vi "ROI entry-bundle parameter values.vi"(7 "XYZ_Coordinates":T1[](array[typedef]) {"ROI group ID" format="%#_6f"; "Laser Power (%)" format="%#_6f"; "Zoom" format="%#_6f"; "Frame Size" format="%#_6f"; "Number of lines" format="%#_6f"; "Composite ID" format="%#_6f"; "Angle (deg)" format="%#_6f"; "ROI Time (ns)" format="%#_6f"; "ROI ID" format="%#_6f"; "Pixels in ROI" format="%#_6f"; "ROI index" format="%#_6f"; "Z stop" format="%#_6f"; "Y stop" format="%#_6f"; "X stop" format="%#_6f"; "Z start" format="%#_6f"; "X start" format="%#_6f"; "Y start" format="%#_6f"}, 8 "error in (no error)":errorcluster, 9 "Button Label.Text":string) -> (0 "error out":errorcluster, 3 "AOL_Globals out":T2={"Imaging Protocol"=enum."AOL Z-Stack", "Number of POI"=0, "Number of Miniscans"=0, "Number of Trials"=0, "Number of Cycles "=0, "# Averaged Frames"=0, "Laser power (%)"=0, "Pockels (V)"=0.0, "Acquisition Length (sec)"=0.0, "Fill time (us)"=0.0, "POI Dwell time (us)"=0.0, "Miniscan Dwell time per pixel (us)"=0.0, "PMT 1"=0.0, "PMT 2"=0.0, "Back Apperture (mA)"=0.0, "Frame Size"=0, "Center Frequency"=0.0, "Field of View (norm)"=0.0, "DwellTime (us)"=0.0, "Wavelength (nm)"=0.0, "Zoom"=0.0, "AOL Z"=0.0, "AOL Mode"=enum."Raster", "GridXY"=0.0, "GridZ"=0.0, "TriggerPeriod (sec)"=0.0, "Number of Pixels in Miniscan"=0, "Experiment folder path"=path "", "X centre"=0.0, "Y centre"=0.0, "Angle (degrees)"=0.0, "Plane Mode"=0, "Threshold"=[], "Regenerate Chirps"=FALSE, "Rectangle ROI length (pixels)"=0, "Rectangle ROI height (pixels)"=0, "AOD fill"=4900, "StartupDelay"=0, "Samples Wait after Trigger"=5080, "Slip Cycle"=600000, "Add Cycle"=TRUE, "Functional Mode"=enum."Point", "Z Start"=0.0, "Z Stop"=0.0, "# Planes"=0} {"Plane Mode" items=["XY Plane", "XZ Plane", "YZ Plane", "arbitraryplane"]; "Frame Size" items=["100X100"=100, "128X128"=128, "200X200"=200, "256X256"=256, "512X512"=512, "1024x1024"=1024, "2048x2048"=2048]; "Back Apperture (mA)" format="%#.6g"; "Pockels (V)" format="%#.6g"; "PMT 2" format="%#.6g"; "PMT 1" format="%#.6g"; "Angle (degrees)" format="%#.6g"; "POI Dwell time (us)" format="%#.6g"})   [LabVIEW 2017]
uses:
  Typedefs/Controls/AOL_Globals.ctl
  Typedefs/Imaging Protocols enum.ctl
  Typedefs/Frame Size.ctl
  Typedefs/AOL modes.ctl
  Typedefs/Plane Mode.ctl
  Typedefs/Functional Mode.ctl
  Visualisation/Functional Imaging Viewer/Typedefs/ROI parameters data type.ctl
  <userlib>/_MGI/Application Control/MGI Change Detector/MGI Change Detector (T).vi
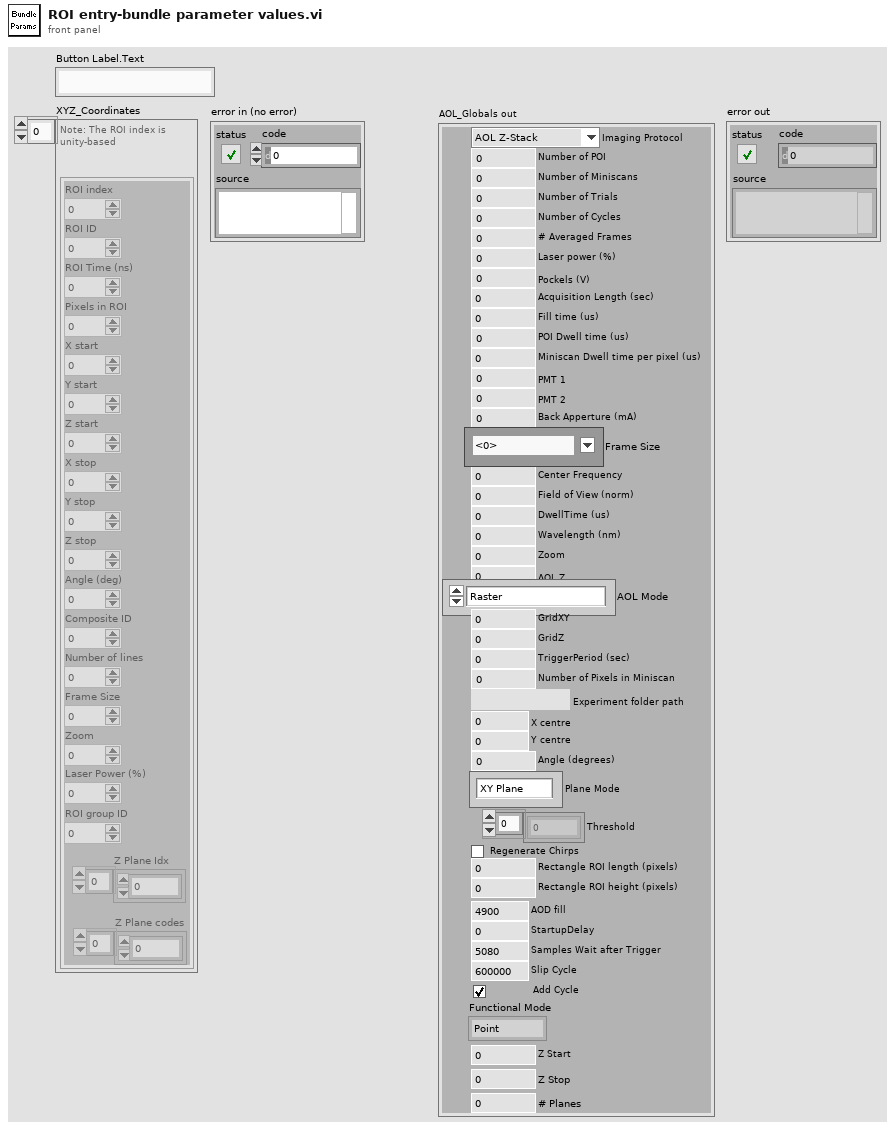
[diagram p1: front panel]
types:
  T1 = typedef "ROI parameters data type.ctl" = cluster{"ROI index":dbl, "ROI ID":dbl, "ROI Time (ns)":dbl, "Pixels in ROI":dbl, "X start":dbl, "Y start":dbl, "Z start":dbl, "X stop":dbl, "Y stop":dbl, "Z stop":dbl, "Angle (deg)":dbl, "Composite ID":dbl, "Number of lines":dbl, "Frame Size":dbl, "Zoom":dbl, "Laser Power (%)":dbl, "ROI group ID":dbl, "Z Plane Idx":i32[], "Z Plane codes":i32[]}
  T2 = typedef "AOL_Globals.ctl" = cluster{"Imaging Protocol":T3, "Number of POI":u16, "Number of Miniscans":u16, "Number of Trials":u16, "Number of Cycles ":u64, "# Averaged Frames":u16, "Laser power (%)":u8, "Pockels (V)":dbl, "Acquisition Length (sec)":dbl, "Fill time (us)":dbl, "POI Dwell time (us)":dbl, "Miniscan Dwell time per pixel (us)":dbl, "PMT 1":dbl, "PMT 2":dbl, "Back Apperture (mA)":dbl, "Frame Size":T4, "Center Frequency":dbl, "Field of View (norm)":dbl, "DwellTime (us)":dbl, "Wavelength (nm)":dbl, "Zoom":dbl, "AOL Z":dbl, "AOL Mode":T5, "GridXY":dbl, "GridZ":dbl, "TriggerPeriod (sec)":dbl, "Number of Pixels in Miniscan":u16, "Experiment folder path":path, "X centre":dbl, "Y centre":dbl, "Angle (degrees)":dbl, "Plane Mode":T6, "Threshold":u16[], "Regenerate Chirps":bool, "Rectangle ROI length (pixels)":u16, "Rectangle ROI height (pixels)":u16, "AOD fill":u16, "StartupDelay":i32, "Samples Wait after Trigger":u16, "Slip Cycle":u32, "Add Cycle":bool, "Functional Mode":T7, "Z Start":dbl, "Z Stop":dbl, "# Planes":i32}
  T3 = typedef "Imaging Protocols enum.ctl" = enum16{"AOL Z-Stack", "Motor Z Stack", "Functional Acquisition", "Single Plane Acquisition", "Volume Acquisition", "Live Imaging", "Live Plane Imaging", "Live Volume Imaging"}
  T4 = typedef "Frame Size.ctl" = u16
  T5 = typedef "AOL modes.ctl" = enum16{"Raster", "Structural", "Pointing", "Mini Scan", "Alignment"}
  T6 = typedef "Plane Mode.ctl" = u16
  T7 = typedef "Functional Mode.ctl" = enum16{"Point", "Line", "Patch", "Plane", "Volume"}
  T8 = typedef "ROI ID Enum.ctl" = enum16{"Point", "MiniScan", "Comp. MiniScan", "Rectangle", "Comp. volume", "Arb. plane point", "None"}
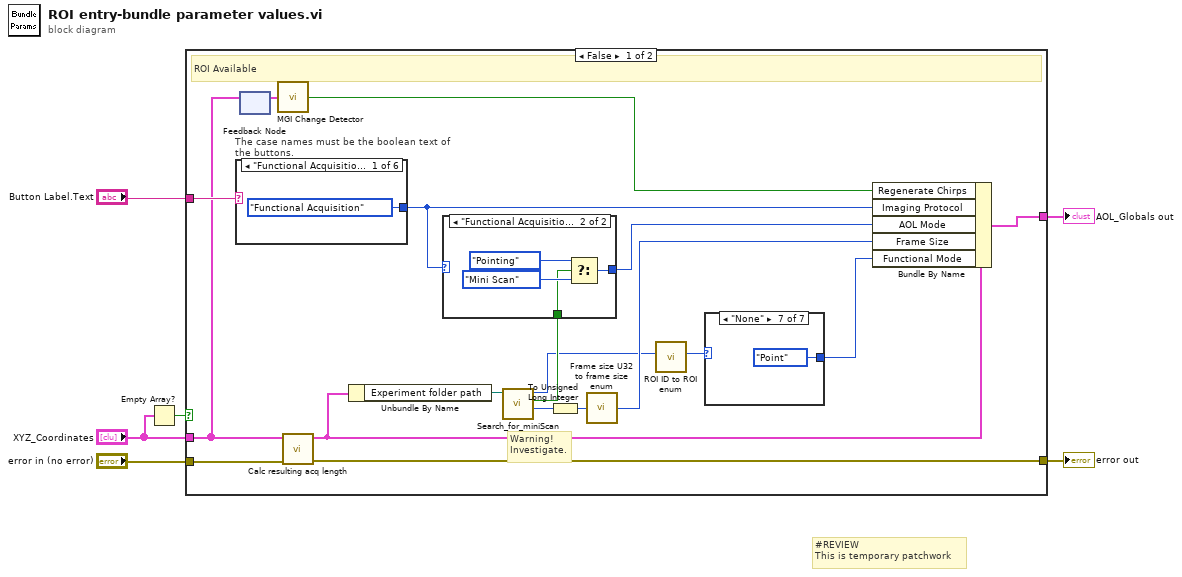
[diagram p0: block diagram]
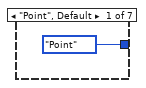
[diagram p2: hidden frame]
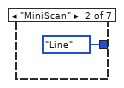
[diagram p3: hidden frame]
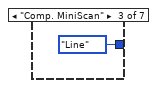
[diagram p4: hidden frame]
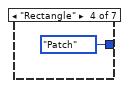
[diagram p5: hidden frame]
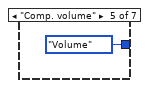
[diagram p6: hidden frame]
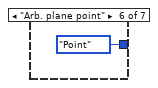
[diagram p7: hidden frame]
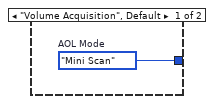
[diagram p8: hidden frame]
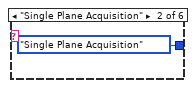
[diagram p9: hidden frame]
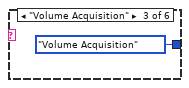
[diagram p10: hidden frame]
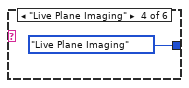
[diagram p11: hidden frame]
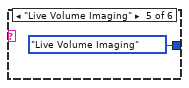
[diagram p12: hidden frame]
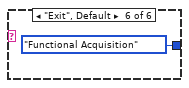
[diagram p13: hidden frame]
diagram:
  # "#REVIEW\nThis is temporary patchwork"
  n1 = Empty Array?(array="XYZ_Coordinates") -> (empty?=w4:bool)
  n2 = case shown="False" w4 {
    tunnel: "XYZ_Coordinates" -> [w12 _]
    tunnel: [w23 _] -> w6
    tunnel: [w22 _] -> w5
    tunnel: "Button Label.Text" -> [w20 _]
    tunnel: "error in (no error)" -> [w18 _]
    frame False {
      # "Warning!\nInvestigate."
      # "ROI Available"
      n3 = case "The case names must be the boolean text of the buttons." shown="\"Functional Acquisition\"" w20 {
        tunnel: [Imaging_Protocols_enum."Functional Acquisition" ("Imaging Protocol") Imaging_Protocols_enum."Single Plane Acquisition" ("Imaging Protocol") Imaging_Protocols_enum."Volume Acquisition" ("Imaging Protocol") Imaging_Protocols_enum."Live Plane Imaging" ("Imaging Protocol") Imaging_Protocols_enum."Live Volume Imaging" ("Imaging Protocol") Imaging_Protocols_enum."Functional Acquisition" ("Imaging Protocol")] -> w19
        frame "Functional Acquisition" {
        }
        frame "Single Plane Acquisition" {
        }
        frame "Volume Acquisition" {
        }
        frame "Live Plane Imaging" {
        }
        frame "Live Volume Imaging" {
        }
        frame "Exit", Default {
        }
      }
      n4 = feedback #1() -> (w24:T1[])  [unwired: 1 in]
      n5 = feedback-in #1(w12) -> ()
      n6 = call-poly <userlib>:"MGI Change Detector.vi"("Value"=w24) -> ("Changed?"=w11:bool)
      n7 = call "Calc resulting acq length.vi"("error in (no error)"=w18, "XYZ_Coordinates"=w12) -> ("error out"=w23:errorcluster, "Output cluster"=w10:T2)  [unwired: 8 in]
      n8 = Unbundle By Name(w10) -> ("Experiment folder path"=w21:path)
      n9 = call "Search_for_miniScan.vi"("AOL ZStack Path"=w21) -> ("Frame Size"=w15:i64, "POI/ROI"=w16:bool, "ROI ID"=w9:i64)  [unwired: 8 in]
      n10 = case shown="\"Functional Acquisition\"" w19 {
        tunnel: [w32 w35] -> w17
        tunnel: w16 -> [_ w34]
        frame "Volume Acquisition", Default {
          w32 = AOL_modes."Mini Scan"  # AOL Mode
        }
        frame "Functional Acquisition" {
          n11 = Select(t=AOL_modes."Pointing" ("AOL Mode"), s=w34, f=AOL_modes."Mini Scan" ("AOL Mode")) -> (s? t:f=w35:T5)
        }
      }
      n12 = To Unsigned Long Integer(number=w15) -> (unsigned 32bit integer=w14:u32)
      n13 = call "Frame size U32 to frame size enum.vi"("Frame Size U32"=w14) -> ("Value"=w13:T4)
      n14 = call "ROI ID to ROI enum.vi"("ROI ID"=w9) -> ("ROI Enum"=w8:T8)  [unwired: 6 in]
      n15 = case shown="\"None\"" w8 {
        tunnel: [Functional_Mode."Point" ("Functional Mode") Functional_Mode."Line" ("Functional Mode") Functional_Mode."Line" ("Functional Mode") Functional_Mode."Patch" ("Functional Mode") Functional_Mode."Volume" ("Functional Mode") Functional_Mode."Point" ("Functional Mode") Functional_Mode."Point" ("Functional Mode")] -> w7
        frame "Point", Default {
        }
        frame "MiniScan" {
        }
        frame "Comp. MiniScan" {
        }
        frame "Rectangle" {
        }
        frame "Comp. volume" {
        }
        frame "Arb. plane point" {
        }
        frame "None" {
        }
      }
      n16 = Bundle By Name(cluster=w10, "Regenerate Chirps"=w11, "Imaging Protocol"=w19, "AOL Mode"=w17, "Frame Size"=w13, "Functional Mode"=w7) -> (w22:T2)
    }
    frame True {
      # "No ROI Entered"
    }
  }
  "AOL_Globals out" <- w5
  "error out" <- w6
